vi "TwChangePeakTableFromFile.vi"(0 "error in (no error)":errorcluster, 1 "filename":string, 4 "compressionLevel":i32) -> (5 "error out":errorcluster)   [LabVIEW 2009]
uses:
  TwH5Dll.dll
panel:
  in  "massTable":string
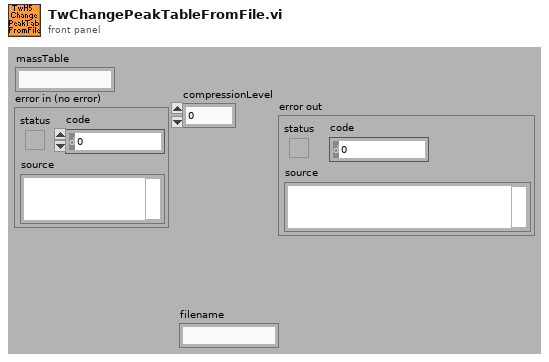
[diagram p1: front panel]
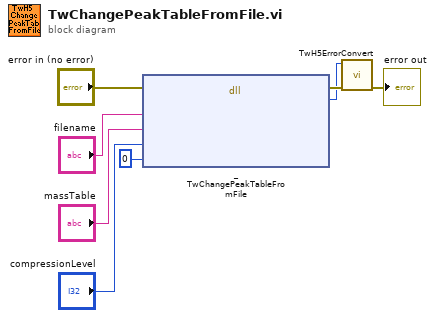
[diagram p0: block diagram]
diagram:
  n1 = dll-call lib="C:/src/85_TofDaq_current/DllWrappers/LabView/TwH5Dll/TwH5Dll.dll" fn="_TwChangePeakTableFromFile"(error in="error in (no error)", "filename"="filename", "massTable"="massTable", "compressionLevel"="compressionLevel", "callback"=u32 0) -> (error out=w7:errorcluster, "TwRetVal"=w6:i32)  [unwired: 5 in, 2 out]
  n2 = call "TwH5ErrorConvert.vi"("error in (no error)"=w7, "error code"=w6) -> ("error out"=→"error out":errorcluster)  [unwired: 9 out]
